vi "myRIO_BRig_RT__Case_Exp_State_initTrial_LC_Sel__v4.vi"(6 "input_dataTrial":u16[][](array[numeric]), 7 "input_spout":enum16{"Left", "Right"}(ring), 8 "input_arrTrig":bool[](array[boolean]), 9 "input_dataBlock":u16[][](array[numeric]), 10 "input_dataLC":u16[](array[numeric]), 11 "input_dataCurrent":u16[](array[numeric])) -> (0 "output_arrTrig":bool[](array[boolean]), 4 "output_dataTrial":u16[][](array[numeric]), 5 "output_dataCurrent":u16[](array[numeric]))   [LabVIEW 2014]
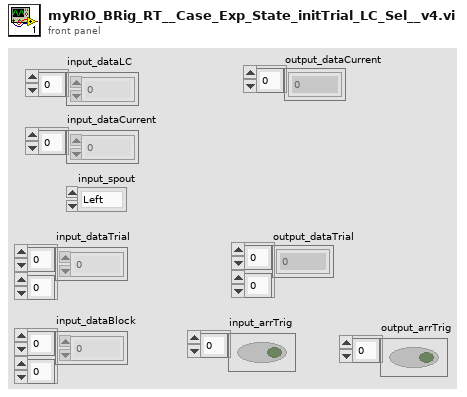
[diagram p1: front panel]
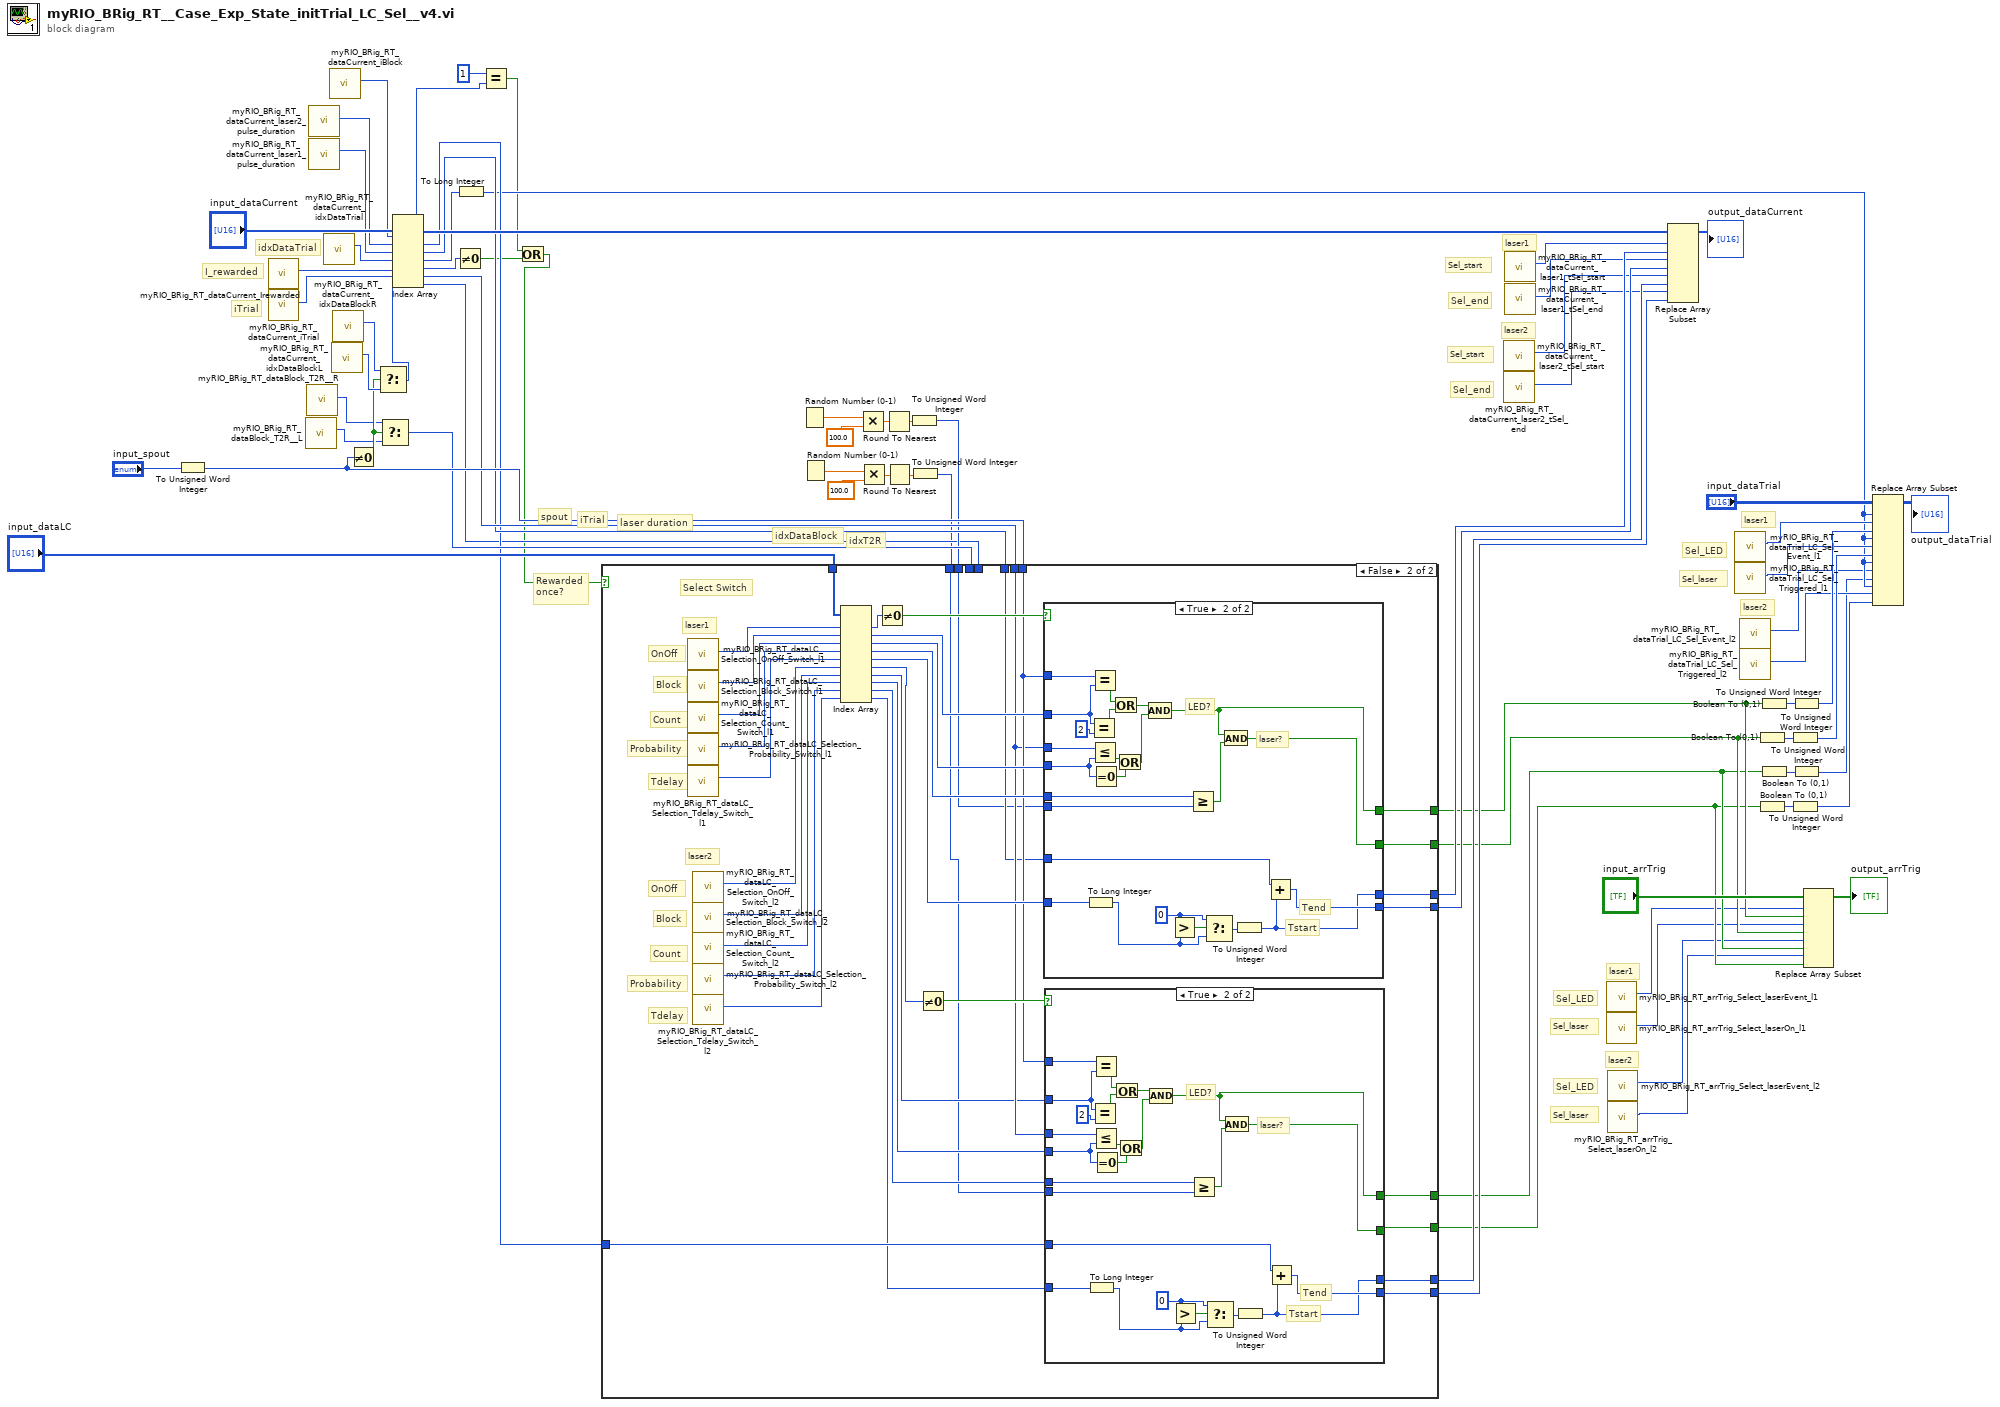
[diagram p0: block diagram]
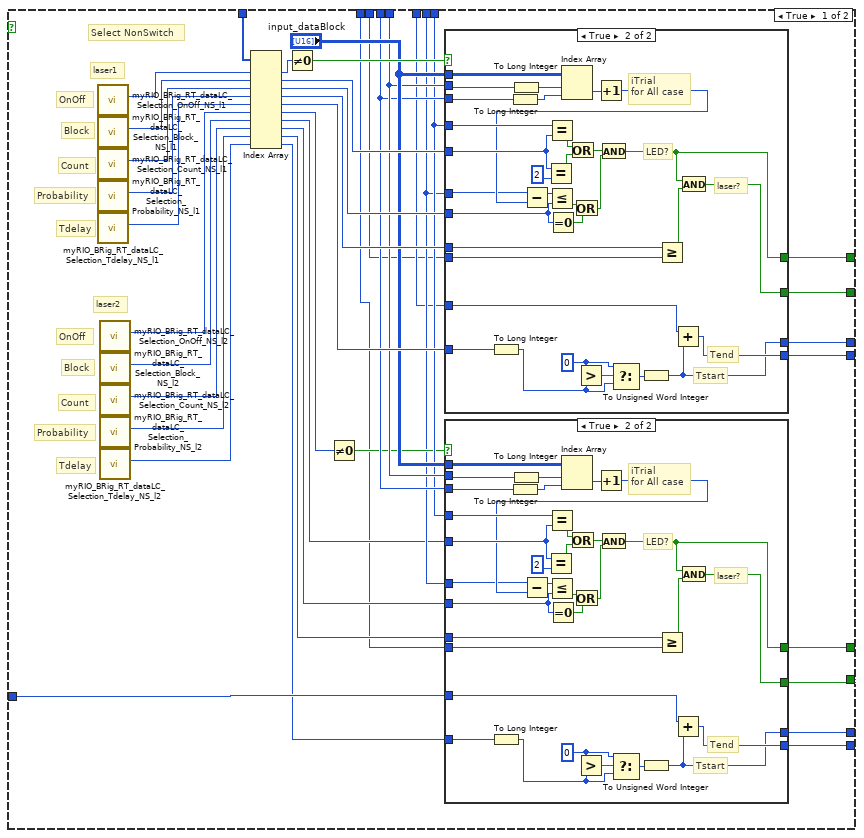
[diagram p2: hidden frame]
diagram:
  # "Sel_LED"
  # "Sel_laser"
  # "Sel_end"
  # "Sel_start"
  # "Sel_LED"
  # "Sel_laser"
  # "Sel_end"
  # "Sel_start"
  # "Sel_LED"
  # "Sel_laser"
  # "laser2"
  # "laser1"
  # "laser2"
  # "laser1"
  # "laser2"
  # "laser1"
  # "idxT2R"
  # "idxDataBlock"
  # "laser duration"
  # "iTrial"
  # "spout"
  # "Rewarded\nonce?"
  # "iTrial"
  # "idxDataTrial"
  # "I_rewarded"
  n1 = To Unsigned Word Integer(number="input_spout") -> (unsigned 16bit integer=w49:u16)
  n2 = call "myRIO_BRig_RT_dataCurrent_Irewarded.vi"() -> ("output_I_rewarded"=w70:i32)  [unwired: 11 in]
  n3 = call "myRIO_BRig_RT_dataCurrent_iTrial.vi"() -> ("output_iTrial"=w59:i32)  [unwired: 11 in]
  n4 = call "myRIO_BRig_RT_dataBlock_T2R__L.vi"() -> ("output_T2R__L"=w54:i32)  [unwired: 11 in]
  n5 = call "myRIO_BRig_RT_dataBlock_T2R__R.vi"() -> ("output_T2R__R"=w55:i32)  [unwired: 11 in]
  n6 = call "myRIO_BRig_RT_dataCurrent_laser2_pulse_duration.vi"() -> ("output_laser2_pulse_duration"=w30:i32)  [unwired: 11 in]
  n7 = call "myRIO_BRig_RT_dataCurrent_laser1_pulse_duration.vi"() -> ("output_laser1_pulse_duration"=w53:i32)  [unwired: 11 in]
  n8 = call "myRIO_BRig_RT_dataCurrent_idxDataTrial.vi"() -> ("output_idxDataTrial"=w63:i32)  [unwired: 11 in]
  n9 = call "myRIO_BRig_RT_dataCurrent_iBlock.vi"() -> ("output_iBlock"=w4:i32)  [unwired: 11 in]
  n10 = call "myRIO_BRig_RT_dataCurrent_idxDataBlockL.vi"() -> ("output_idxDataBlock__L"=w58:i32)  [unwired: 11 in]
  n11 = call "myRIO_BRig_RT_dataCurrent_idxDataBlockR.vi"() -> ("output_idxDataBlock__R"=w57:i32)  [unwired: 11 in]
  n12 = Not Equal To 0?(x=w49) -> (x != 0?=w56:bool)
  n13 = Select(t=w57, s=w56, f=w58) -> (s? t:f=w27:i32)
  n14 = Select(t=w55, s=w56, f=w54) -> (s? t:f=w46:i32)
  n15 = Index Array(array="input_dataCurrent", index #1=w4, index #2=w30, index #3=w53, index #4=w63, index #5=w70, index #6=w59, index #7=w27) -> (element #1=w3:u16, element #2=w29:u16, element #3=w47:u16, element #4=w62:u16, element #5=w71:u16, element #6=w48:u16, element #7=w28:u16)
  n16 = Not Equal To 0?(x=w71) -> (x != 0?=w2:bool)
  n17 = To Long Integer(number=w62) -> (32bit integer=w16:i32)
  n18 = Equal?(x=u16 1, y=w3) -> (x = y?=w5:bool)
  n19 = Or(x=w5, y=w2) -> (x .or. y?=w1:bool)
  n20 = Random Number (0-1)() -> (number: 0 to 1=w42:dbl)
  n21 = Random Number (0-1)() -> (number: 0 to 1=w8:dbl)
  n22 = Multiply(x=w42, y=100.0) -> (x*y=w43:dbl)
  n23 = Multiply(x=w8, y=100.0) -> (x*y=w9:dbl)
  n24 = Round To Nearest(number=w43) -> (nearest integer value=w44:dbl)
  n25 = Round To Nearest(number=w9) -> (nearest integer value=w10:dbl)
  n26 = To Unsigned Word Integer(number=w44) -> (unsigned 16bit integer=w41:u16)
  n27 = To Unsigned Word Integer(number=w10) -> (unsigned 16bit integer=w7:u16)
  n28 = case shown="False" w1 {
    tunnel: "input_dataLC" -> [w112 w213]
    tunnel: w49 -> [w102 w197]
    tunnel: w48 -> [w100 w196]
    tunnel: w47 -> [w99 w195]
    tunnel: w28 -> [w104 _]
    tunnel: w46 -> [w103 _]
    tunnel: w41 -> [w73 w177]
    tunnel: [w98 w206] -> w34
    tunnel: [w97 w205] -> w33
    tunnel: [w96 w204] -> w40
    tunnel: [w95 w203] -> w39
    tunnel: [w94 w201] -> w32
    tunnel: [w93 w200] -> w31
    tunnel: [w92 w199] -> w38
    tunnel: [w91 w198] -> w37
    tunnel: w29 -> [w90 w194]
    tunnel: w7 -> [w74 w178]
    frame True {
      # "laser2"
      # "laser1"
      # "Count"
      # "Tdelay"
      # "Probability"
      # "OnOff"
      # "Block"
      # "Count"
      # "Tdelay"
      # "Probability"
      # "OnOff"
      # "Block"
      # "Select NonSwitch"
      n29 = call "myRIO_BRig_RT_dataLC_Selection_OnOff_NS_l1.vi"() -> ("output_Selection_OnOff_NS_l1"=w75:i32)  [unwired: 11 in]
      n30 = call "myRIO_BRig_RT_dataLC_Selection_Block_NS_l1.vi"() -> ("output_Selection_Block_NS_l1"=w76:i32)  [unwired: 11 in]
      n31 = call "myRIO_BRig_RT_dataLC_Selection_Count_NS_l1.vi"() -> ("output_Selection_Count_NS_l1"=w77:i32)  [unwired: 11 in]
      n32 = call "myRIO_BRig_RT_dataLC_Selection_Probability_NS_l1.vi"() -> ("output_Selection_Probability_NS_l1"=w78:i32)  [unwired: 11 in]
      n33 = call "myRIO_BRig_RT_dataLC_Selection_Tdelay_NS_l1.vi"() -> ("output_Selection_Tdelay_NS_l1"=w79:i32)  [unwired: 11 in]
      n34 = call "myRIO_BRig_RT_dataLC_Selection_OnOff_NS_l2.vi"() -> ("output_Selection_OnOff_NS_l2"=w84:i32)  [unwired: 11 in]
      n35 = call "myRIO_BRig_RT_dataLC_Selection_Block_NS_l2.vi"() -> ("output_Selection_Block_NS_l2"=w83:i32)  [unwired: 11 in]
      n36 = call "myRIO_BRig_RT_dataLC_Selection_Count_NS_l2.vi"() -> ("output_Selection_Count_NS_l2"=w82:i32)  [unwired: 11 in]
      n37 = call "myRIO_BRig_RT_dataLC_Selection_Probability_NS_l2.vi"() -> ("output_Selection_Probability_NS_l2"=w81:i32)  [unwired: 11 in]
      n38 = call "myRIO_BRig_RT_dataLC_Selection_Tdelay_NS_l2.vi"() -> ("output_Selection_Tdelay_NS_l2"=w80:i32)  [unwired: 11 in]
      n39 = Index Array(array=w112, index #1=w75, index #2=w76, index #3=w77, index #4=w78, index #5=w79, index #6=w84, index #7=w83, index #8=w82, index #9=w81, index #10=w80) -> (element #1=w108:u16, element #2=w106:u16, element #3=w111:u16, element #4=w110:u16, element #5=w109:u16, element #6=w89:u16, element #7=w88:u16, element #8=w87:u16, element #9=w86:u16, element #10=w85:u16)
      n40 = Not Equal To 0?(x=w108) -> (x != 0?=w107:bool)
      n41 = Not Equal To 0?(x=w89) -> (x != 0?=w101:bool)
      n42 = case shown="True" w107 {
        tunnel: w102 -> [_ w175]
        tunnel: w100 -> [_ w160]
        tunnel: [_ w155] -> w98
        tunnel: [_ w171] -> w97
        tunnel: [_ w151] -> w95
        tunnel: [_ w150] -> w96
        tunnel: w99 -> [_ w149]
        tunnel: w103 -> [_ w166]
        tunnel: w104 -> [_ w168]
        tunnel: w106 -> [_ w163]
        tunnel: w111 -> [_ w162]
        tunnel: w110 -> [_ w158]
        tunnel: w109 -> [_ w148]
        tunnel: "input_dataBlock" -> [_ w147]
        tunnel: w73 -> [_ w146]
        frame False {
        }
        frame True {
          w153 = 0 ("x")
          # "Tstart"
          # "Tend"
          # "iTrial\nfor All case"
          # "laser?"
          # "LED?"
          n43 = To Long Integer(number=w148) -> (32bit integer=w145:i32)
          n44 = To Long Integer(number=w166) -> (32bit integer=w165:i32)
          n45 = To Long Integer(number=w168) -> (32bit integer=w167:i32)
          n46 = Equal?(x=w163, y=u16 2) -> (x = y?=w173:bool)
          n47 = Equal?(x=w175, y=w163) -> (x = y?=w174:bool)
          n48 = Equal To 0?(x=w162) -> (x = 0?=w169:bool)
          n49 = Index Array(array=w147, index (row)=w167, index (col)=w165) -> (element=w164:u16)
          n50 = Or(x=w174, y=w173) -> (x .or. y?=w157:bool)
          n51 = Greater?(x=w153, y=w145) -> (0:w152:bool)
          n52 = Increment(x=w164) -> (x+1=w161:u16)
          n53 = Subtract(x=w160, y=w161) -> (x-y=w159:u16)
          n54 = Less Or Equal?(x=w159, y=w162) -> (x <= y?=w170:bool)
          n55 = Or(x=w170, y=w169) -> (x .or. y?=w156:bool)
          n56 = And(x=w157, y=w156) -> (x .and. y?=w155:bool)
          n57 = Select(t=w153, s=w152, f=w145) -> (s? t:f=w154:i32)
          n58 = To Unsigned Word Integer(number=w154) -> (unsigned 16bit integer=w150:u16)
          n59 = Greater Or Equal?(x=w158, y=w146) -> (x >= y?=w172:bool)
          n60 = Add(x=w149, y=w150) -> (x+y=w151:u16)
          n61 = And(x=w155, y=w172) -> (x .and. y?=w171:bool)
        }
      }
      n62 = case shown="True" w101 {
        tunnel: w102 -> [_ w143]
        tunnel: w100 -> [_ w128]
        tunnel: [_ w123] -> w94
        tunnel: [_ w139] -> w93
        tunnel: [_ w119] -> w91
        tunnel: [_ w118] -> w92
        tunnel: w90 -> [_ w117]
        tunnel: w103 -> [_ w134]
        tunnel: w104 -> [_ w136]
        tunnel: w88 -> [_ w131]
        tunnel: w87 -> [_ w130]
        tunnel: w86 -> [_ w126]
        tunnel: w85 -> [_ w116]
        tunnel: "input_dataBlock" -> [_ w115]
        tunnel: w74 -> [_ w114]
        frame False {
        }
        frame True {
          w121 = 0 ("x")
          # "Tstart"
          # "Tend"
          # "iTrial\nfor All case"
          # "laser?"
          # "LED?"
          n63 = To Long Integer(number=w116) -> (32bit integer=w113:i32)
          n64 = To Long Integer(number=w134) -> (32bit integer=w133:i32)
          n65 = To Long Integer(number=w136) -> (32bit integer=w135:i32)
          n66 = Equal?(x=w131, y=u16 2) -> (x = y?=w141:bool)
          n67 = Equal?(x=w143, y=w131) -> (x = y?=w142:bool)
          n68 = Equal To 0?(x=w130) -> (x = 0?=w137:bool)
          n69 = Index Array(array=w115, index (row)=w135, index (col)=w133) -> (element=w132:u16)
          n70 = Or(x=w142, y=w141) -> (x .or. y?=w125:bool)
          n71 = Greater?(x=w121, y=w113) -> (0:w120:bool)
          n72 = Increment(x=w132) -> (x+1=w129:u16)
          n73 = Subtract(x=w128, y=w129) -> (x-y=w127:u16)
          n74 = Less Or Equal?(x=w127, y=w130) -> (x <= y?=w138:bool)
          n75 = Or(x=w138, y=w137) -> (x .or. y?=w124:bool)
          n76 = And(x=w125, y=w124) -> (x .and. y?=w123:bool)
          n77 = Select(t=w121, s=w120, f=w113) -> (s? t:f=w122:i32)
          n78 = To Unsigned Word Integer(number=w122) -> (unsigned 16bit integer=w118:u16)
          n79 = Greater Or Equal?(x=w126, y=w114) -> (x >= y?=w140:bool)
          n80 = Add(x=w117, y=w118) -> (x+y=w119:u16)
          n81 = And(x=w123, y=w140) -> (x .and. y?=w139:bool)
        }
      }
    }
    frame False {
      # "laser2"
      # "laser1"
      # "Count"
      # "Tdelay"
      # "Probability"
      # "OnOff"
      # "Block"
      # "Count"
      # "Tdelay"
      # "Probability"
      # "OnOff"
      # "Block"
      # "Select Switch"
      n82 = call "myRIO_BRig_RT_dataLC_Selection_OnOff_Switch_l1.vi"() -> ("output_Selection_OnOff_Switch_l1"=w193:i32)  [unwired: 11 in]
      n83 = call "myRIO_BRig_RT_dataLC_Selection_Block_Switch_l1.vi"() -> ("output_Selection_Block_Switch_l1"=w192:i32)  [unwired: 11 in]
      n84 = call "myRIO_BRig_RT_dataLC_Selection_Count_Switch_l1.vi"() -> ("output_Selection_Count_Switch_l1"=w191:i32)  [unwired: 11 in]
      n85 = call "myRIO_BRig_RT_dataLC_Selection_Probability_Switch_l1.vi"() -> ("output_Selection_Probability_Switch_l1"=w190:i32)  [unwired: 11 in]
      n86 = call "myRIO_BRig_RT_dataLC_Selection_Tdelay_Switch_l1.vi"() -> ("output_Selection_Tdelay_Switch_l1"=w189:i32)  [unwired: 11 in]
      n87 = call "myRIO_BRig_RT_dataLC_Selection_OnOff_Switch_l2.vi"() -> ("output_Selection_OnOff_Switch_l2"=w179:i32)  [unwired: 11 in]
      n88 = call "myRIO_BRig_RT_dataLC_Selection_Block_Switch_l2.vi"() -> ("output_Selection_Block_Switch_l2"=w180:i32)  [unwired: 11 in]
      n89 = call "myRIO_BRig_RT_dataLC_Selection_Count_Switch_l2.vi"() -> ("output_Selection_Count_Switch_l2"=w181:i32)  [unwired: 11 in]
      n90 = call "myRIO_BRig_RT_dataLC_Selection_Probability_Switch_l2.vi"() -> ("output_Selection_Probability_Switch_l1"=w182:i32)  [unwired: 11 in]
      n91 = call "myRIO_BRig_RT_dataLC_Selection_Tdelay_Switch_l2.vi"() -> ("output_Selection_Tdelay_Switch_l2"=w183:i32)  [unwired: 11 in]
      n92 = Index Array(array=w213, index #1=w193, index #2=w192, index #3=w191, index #4=w190, index #5=w189, index #6=w179, index #7=w180, index #8=w181, index #9=w182, index #10=w183) -> (element #1=w212:u16, element #2=w209:u16, element #3=w208:u16, element #4=w210:u16, element #5=w207:u16, element #6=w188:u16, element #7=w187:u16, element #8=w186:u16, element #9=w185:u16, element #10=w184:u16)
      n93 = Not Equal To 0?(x=w212) -> (x != 0?=w211:bool)
      n94 = Not Equal To 0?(x=w188) -> (x != 0?=w202:bool)
      n95 = case shown="True" w211 {
        tunnel: w197 -> [_ w260]
        tunnel: w209 -> [_ w259]
        tunnel: w196 -> [_ w258]
        tunnel: [_ w253] -> w206
        tunnel: [_ w252] -> w205
        tunnel: [_ w242] -> w203
        tunnel: w207 -> [_ w244]
        tunnel: [_ w241] -> w204
        tunnel: w208 -> [_ w251]
        tunnel: w195 -> [_ w243]
        tunnel: w177 -> [_ w240]
        tunnel: w210 -> [_ w239]
        frame False {
        }
        frame True {
          w246 = 0 ("x")
          # "Tstart"
          # "Tend"
          # "laser?"
          # "LED?"
          n96 = To Long Integer(number=w244) -> (32bit integer=w238:i32)
          n97 = Equal?(x=w259, y=u16 2) -> (x = y?=w256:bool)
          n98 = Equal?(x=w260, y=w259) -> (x = y?=w257:bool)
          n99 = Less Or Equal?(x=w258, y=w251) -> (x <= y?=w250:bool)
          n100 = Equal To 0?(x=w251) -> (x = 0?=w249:bool)
          n101 = Or(x=w257, y=w256) -> (x .or. y?=w255:bool)
          n102 = Or(x=w250, y=w249) -> (x .or. y?=w248:bool)
          n103 = Compound Arithmetic op=AND(w255, w248) -> (w253:bool)
          n104 = Greater?(x=w246, y=w238) -> (0:w245:bool)
          n105 = Greater Or Equal?(x=w239, y=w240) -> (x >= y?=w254:bool)
          n106 = Select(t=w246, s=w245, f=w238) -> (s? t:f=w247:i32)
          n107 = And(x=w253, y=w254) -> (x .and. y?=w252:bool)
          n108 = To Unsigned Word Integer(number=w247) -> (unsigned 16bit integer=w241:u16)
          n109 = Add(x=w243, y=w241) -> (x+y=w242:u16)
        }
      }
      n110 = case shown="True" w202 {
        tunnel: w197 -> [_ w236]
        tunnel: w187 -> [_ w235]
        tunnel: w196 -> [_ w234]
        tunnel: [_ w229] -> w201
        tunnel: [_ w228] -> w200
        tunnel: [_ w218] -> w198
        tunnel: w184 -> [_ w220]
        tunnel: [_ w217] -> w199
        tunnel: w186 -> [_ w227]
        tunnel: w194 -> [_ w219]
        tunnel: w178 -> [_ w216]
        tunnel: w185 -> [_ w215]
        frame False {
        }
        frame True {
          w222 = 0 ("x")
          # "Tstart"
          # "Tend"
          # "laser?"
          # "LED?"
          n111 = To Long Integer(number=w220) -> (32bit integer=w214:i32)
          n112 = Equal?(x=w235, y=u16 2) -> (x = y?=w232:bool)
          n113 = Equal?(x=w236, y=w235) -> (x = y?=w233:bool)
          n114 = Less Or Equal?(x=w234, y=w227) -> (x <= y?=w226:bool)
          n115 = Equal To 0?(x=w227) -> (x = 0?=w225:bool)
          n116 = Or(x=w233, y=w232) -> (x .or. y?=w231:bool)
          n117 = Or(x=w226, y=w225) -> (x .or. y?=w224:bool)
          n118 = Compound Arithmetic op=AND(w231, w224) -> (w229:bool)
          n119 = Greater?(x=w222, y=w214) -> (0:w221:bool)
          n120 = Greater Or Equal?(x=w215, y=w216) -> (x >= y?=w230:bool)
          n121 = Select(t=w222, s=w221, f=w214) -> (s? t:f=w223:i32)
          n122 = And(x=w229, y=w230) -> (x .and. y?=w228:bool)
          n123 = To Unsigned Word Integer(number=w223) -> (unsigned 16bit integer=w217:u16)
          n124 = Add(x=w219, y=w217) -> (x+y=w218:u16)
        }
      }
    }
  }
  n125 = call "myRIO_BRig_RT_dataCurrent_laser2_tSel_start.vi"() -> ("output_laser2_tSel_start"=w24:i32)  [unwired: 11 in]
  n126 = call "myRIO_BRig_RT_dataCurrent_laser2_tSel_end.vi"() -> ("output_laser2_tSel_end"=w23:i32)  [unwired: 11 in]
  n127 = call "myRIO_BRig_RT_dataCurrent_laser1_tSel_start.vi"() -> ("output_laser1_tSel_start"=w25:i32)  [unwired: 11 in]
  n128 = call "myRIO_BRig_RT_dataCurrent_laser1_tSel_end.vi"() -> ("output_laser1_tSel_end"=w26:i32)  [unwired: 11 in]
  n129 = call "myRIO_BRig_RT_arrTrig_Select_laserEvent_l1.vi"() -> ("output_arrTrig_Select_laserEvent_l1"=w21:i32)  [unwired: 11 in]
  n130 = call "myRIO_BRig_RT_arrTrig_Select_laserOn_l1.vi"() -> ("output_arrTrig_Select_laserOn_l1"=w22:i32)  [unwired: 11 in]
  n131 = call "myRIO_BRig_RT_arrTrig_Select_laserEvent_l2.vi"() -> ("output_arrTrig_Select_laserEvent_l2"=w20:i32)  [unwired: 11 in]
  n132 = call "myRIO_BRig_RT_arrTrig_Select_laserOn_l2.vi"() -> ("output_arrTrig_Select_laserOn_l2"=w19:i32)  [unwired: 11 in]
  n133 = Replace Array Subset(array="input_dataCurrent", new element #1=w40, index #1=w25, new element #2=w39, index #2=w26, new element #3=w38, index #3=w24, new element #4=w37, index #4=w23) -> (→"output_dataCurrent":u16[])
  n134 = call "myRIO_BRig_RT_dataTrial_LC_Sel_Event_l1.vi"() -> ("output_LC_Sel_Event_l1"=w17:i32)  [unwired: 11 in]
  n135 = call "myRIO_BRig_RT_dataTrial_LC_Sel_Triggered_l1.vi"() -> ("output_LC_Sel_Triggered_l1"=w18:i32)  [unwired: 11 in]
  n136 = call "myRIO_BRig_RT_dataTrial_LC_Sel_Event_l2.vi"() -> ("output_LC_Sel_Event_l2"=w15:i32)  [unwired: 11 in]
  n137 = call "myRIO_BRig_RT_dataTrial_LC_Sel_Triggered_l2.vi"() -> ("output_LC_Sel_Triggered_l2"=w14:i32)  [unwired: 11 in]
  n138 = Boolean To (0,1)(Boolean=w33) -> (0, 1=w66:i16)
  n139 = Boolean To (0,1)(Boolean=w31) -> (0, 1=w36:i16)
  n140 = Boolean To (0,1)(Boolean=w34) -> (0, 1=w67:i16)
  n141 = Boolean To (0,1)(Boolean=w32) -> (0, 1=w35:i16)
  n142 = To Unsigned Word Integer(number=w66) -> (unsigned 16bit integer=w60:u16)
  n143 = To Unsigned Word Integer(number=w36) -> (unsigned 16bit integer=w12:u16)
  n144 = To Unsigned Word Integer(number=w67) -> (unsigned 16bit integer=w61:u16)
  n145 = To Unsigned Word Integer(number=w35) -> (unsigned 16bit integer=w13:u16)
  n146 = Replace Array Subset(array="input_arrTrig", new element #1=w34, index #1=w21, new element #2=w33, index #2=w22, new element #3=w32, index #3=w20, new element #4=w31, index #4=w19) -> (→"output_arrTrig":bool[])
  n147 = Replace Array Subset(array="input_dataTrial", new element #1=w61, index (row) #1=w16, index (col) #1=w17, new element #2=w60, index (row) #2=w16, index (col) #2=w18, new element #3=w13, index (row) #3=w16, index (col) #3=w15, new element #4=w12, index (row) #4=w16, index (col) #4=w14) -> (→"output_dataTrial":u16[][])
